vi "DatabaseToSharedVariable.vi"(8 "error in":errorcluster, 9 "database":string[][](array[string]), 11 "Library in":refnum<vi>) -> (0 "error out":errorcluster, 2 "Boolean":bool, 3 "Library out":refnum<vi>)   [LabVIEW 2014]
doc: "<B>Copyright</B>: (c) 2015 MHWirth. All rights reserved.\n\nThis subVI creates and addes shared variables to the given library. \nTo generate shared variables, it requires a 2D array of strings, whose first column contains the names and the second one contains the data type.\n\n<B>Limitation</B>: Not available in Run-time Engine."
panel:
  out "Numeric":i32
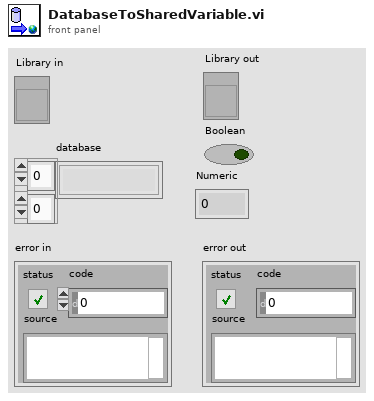
[diagram p1: front panel]
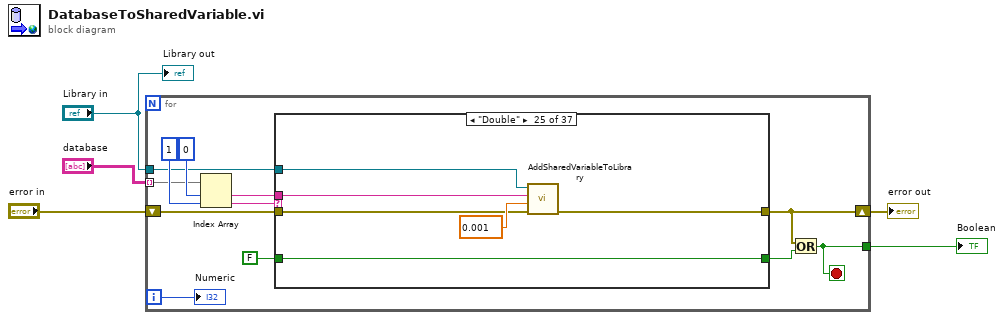
[diagram p0: block diagram]
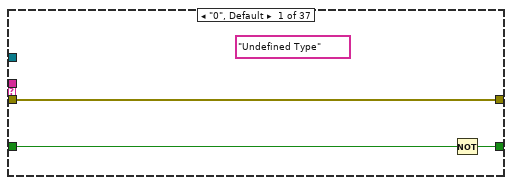
[diagram p2: hidden frame]
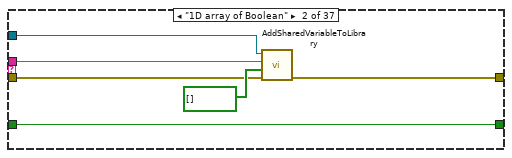
[diagram p3: hidden frame]
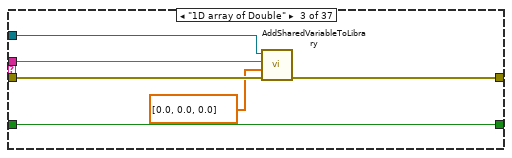
[diagram p4: hidden frame]
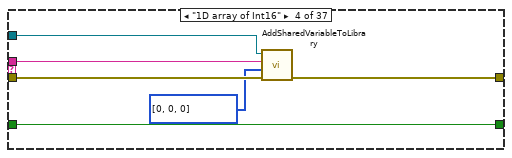
[diagram p5: hidden frame]
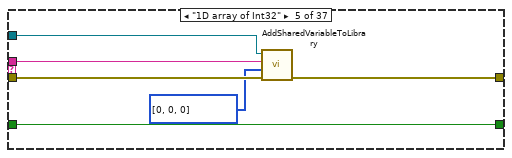
[diagram p6: hidden frame]
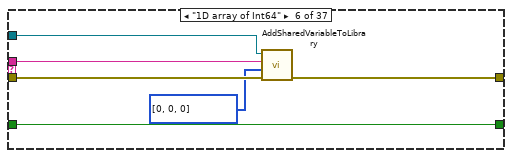
[diagram p7: hidden frame]
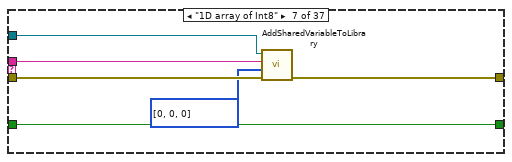
[diagram p8: hidden frame]
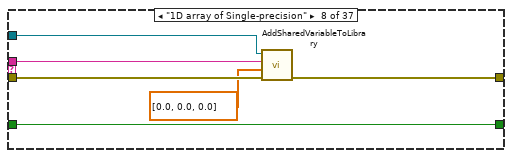
[diagram p9: hidden frame]
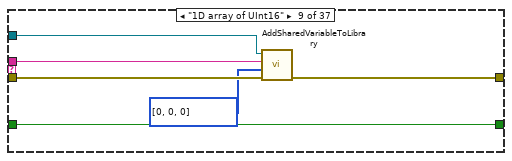
[diagram p10: hidden frame]
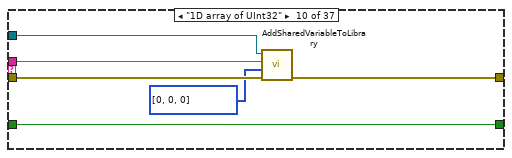
[diagram p11: hidden frame]
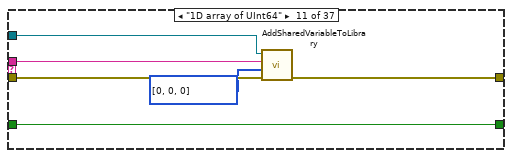
[diagram p12: hidden frame]
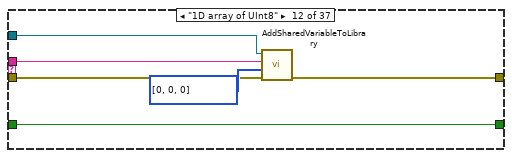
[diagram p13: hidden frame]
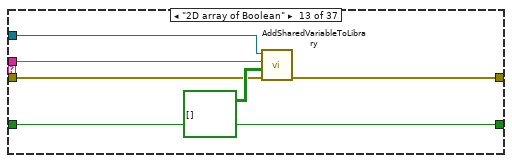
[diagram p14: hidden frame]
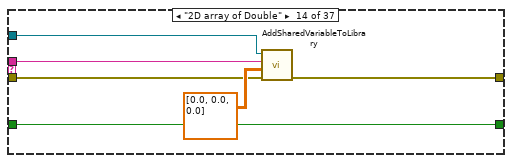
[diagram p15: hidden frame]
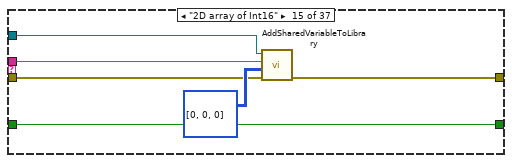
[diagram p16: hidden frame]
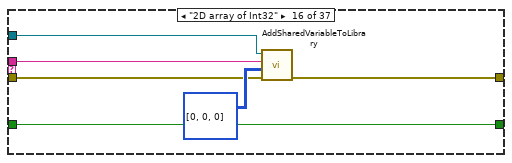
[diagram p17: hidden frame]
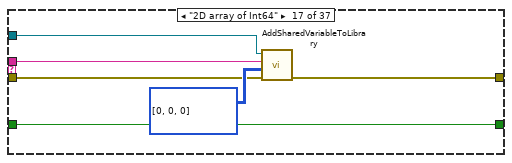
[diagram p18: hidden frame]
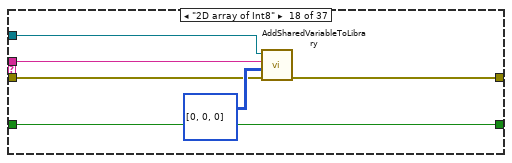
[diagram p19: hidden frame]
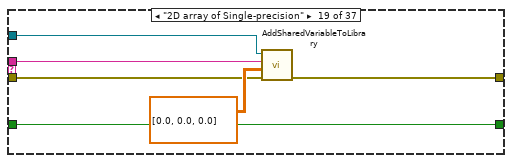
[diagram p20: hidden frame]
diagram:
  n1 = for {
    shift-right: [w7] -> w5
    shift-left: "error in" -> [w8]
    tunnel: "database" -> [w15] mode=indexing
    tunnel: [w11] -> w4
    tunnel: "Library in" -> [w9]
    i -> [w6]
    stop <- w11 stop-if-true
    n2 = Index Array(array=w15, index #1=0 ("index"), index #2=1 ("index")) -> (element #1=w10:string, element #2=w14:string)
    n3 = case shown="\"Double\"" w14 {
      tunnel: FALSE -> [w20 w26 w32 w38 w44 w50 w56 w62 w68 w74 w80 w86 w92 w98 w104 w110 w116 w122 w128 w134 w140 w146 w152 w158 w164 w170 w176 w182 w188 w194 w200 w206 w212 w218 w224 w230 w236]
      tunnel: [w19 w26 w32 w38 w44 w50 w56 w62 w68 w74 w80 w86 w92 w98 w104 w110 w116 w122 w128 w134 w140 w146 w152 w158 w164 w170 w176 w182 w188 w194 w200 w206 w212 w218 w224 w230 w236] -> w12
      tunnel: w10 -> [_ w25 w29 w34 w40 w47 w52 w58 w64 w70 w76 w82 w90 w95 w102 w108 w114 w120 w126 w131 w138 w144 w150 w156 w162 w167 w172 w180 w186 w192 w198 w204 w210 w216 w222 w228 w234]
      tunnel: w9 -> [_ w23 w28 w35 w43 w48 w51 w57 w65 w71 w75 w84 w91 w96 w103 w109 w115 w121 w127 w132 w139 w145 w151 w157 w163 w168 w173 w181 w187 w193 w199 w205 w211 w217 w223 w229 w235]
      tunnel: w8 -> [w18 w22 w30 w36 w42 w49 w54 w60 w66 w72 w78 w83 w88 w93 w100 w106 w112 w118 w124 w133 w136 w142 w148 w154 w160 w166 w174 w178 w184 w190 w196 w202 w208 w214 w220 w226 w232]
      tunnel: [w18 w21 w31 w37 w41 w45 w55 w61 w67 w73 w79 w81 w87 w97 w99 w105 w111 w117 w123 w129 w135 w141 w147 w153 w159 w165 w175 w177 w183 w189 w195 w201 w207 w213 w219 w225 w231] -> w7
      frame "0", Default {
        (unwired) "Undefined Type"
        n4 = Not(x=w20) -> (.not. x?=w19:bool)
      }
      frame "1D array of Boolean" {
        n5 = call <vilib>:"AddSharedVariableToLibrary.vi"("error in (no error)"=w22, "Variable Data Type (Double)"=bool[] [], "Variable Name"=w25, "Library Reference In"=w23) -> ("error out"=w21:errorcluster)  [unwired: 5 in, 2 out]
      }
      frame "1D array of Double" {
        n6 = call <vilib>:"AddSharedVariableToLibrary.vi"("error in (no error)"=w30, "Variable Data Type (Double)"=dbl[] [0.0, 0.0, 0.0], "Variable Name"=w29, "Library Reference In"=w28) -> ("error out"=w31:errorcluster)  [unwired: 5 in, 2 out]
      }
      frame "1D array of Int16" {
        n7 = call <vilib>:"AddSharedVariableToLibrary.vi"("error in (no error)"=w36, "Variable Data Type (Double)"=i16[] [0, 0, 0], "Variable Name"=w34, "Library Reference In"=w35) -> ("error out"=w37:errorcluster)  [unwired: 5 in, 2 out]
      }
      frame "1D array of Int32" {
        n8 = call <vilib>:"AddSharedVariableToLibrary.vi"("error in (no error)"=w42, "Variable Data Type (Double)"=i32[] [0, 0, 0], "Variable Name"=w40, "Library Reference In"=w43) -> ("error out"=w41:errorcluster)  [unwired: 5 in, 2 out]
      }
      frame "1D array of Int64" {
        n9 = call <vilib>:"AddSharedVariableToLibrary.vi"("error in (no error)"=w49, "Variable Data Type (Double)"=i64[] [0, 0, 0], "Variable Name"=w47, "Library Reference In"=w48) -> ("error out"=w45:errorcluster)  [unwired: 5 in, 2 out]
      }
      frame "1D array of Int8" {
        n10 = call <vilib>:"AddSharedVariableToLibrary.vi"("error in (no error)"=w54, "Variable Data Type (Double)"=i8[] [0, 0, 0], "Variable Name"=w52, "Library Reference In"=w51) -> ("error out"=w55:errorcluster)  [unwired: 5 in, 2 out]
      }
      frame "1D array of Single-precision" {
        n11 = call <vilib>:"AddSharedVariableToLibrary.vi"("error in (no error)"=w60, "Variable Data Type (Double)"=sgl[] [0.0, 0.0, 0.0], "Variable Name"=w58, "Library Reference In"=w57) -> ("error out"=w61:errorcluster)  [unwired: 5 in, 2 out]
      }
      frame "1D array of UInt16" {
        n12 = call <vilib>:"AddSharedVariableToLibrary.vi"("error in (no error)"=w66, "Variable Data Type (Double)"=u16[] [0, 0, 0], "Variable Name"=w64, "Library Reference In"=w65) -> ("error out"=w67:errorcluster)  [unwired: 5 in, 2 out]
      }
      frame "1D array of UInt32" {
        n13 = call <vilib>:"AddSharedVariableToLibrary.vi"("error in (no error)"=w72, "Variable Data Type (Double)"=u32[] [0, 0, 0], "Variable Name"=w70, "Library Reference In"=w71) -> ("error out"=w73:errorcluster)  [unwired: 5 in, 2 out]
      }
      frame "1D array of UInt64" {
        n14 = call <vilib>:"AddSharedVariableToLibrary.vi"("error in (no error)"=w78, "Variable Data Type (Double)"=u64[] [0, 0, 0], "Variable Name"=w76, "Library Reference In"=w75) -> ("error out"=w79:errorcluster)  [unwired: 5 in, 2 out]
      }
      frame "1D array of UInt8" {
        n15 = call <vilib>:"AddSharedVariableToLibrary.vi"("error in (no error)"=w83, "Variable Data Type (Double)"=u8[] [0, 0, 0], "Variable Name"=w82, "Library Reference In"=w84) -> ("error out"=w81:errorcluster)  [unwired: 5 in, 2 out]
      }
      frame "2D array of Boolean" {
        n16 = call <vilib>:"AddSharedVariableToLibrary.vi"("error in (no error)"=w88, "Variable Data Type (Double)"=bool[][] [], "Variable Name"=w90, "Library Reference In"=w91) -> ("error out"=w87:errorcluster)  [unwired: 5 in, 2 out]
      }
      frame "2D array of Double" {
        n17 = call <vilib>:"AddSharedVariableToLibrary.vi"("error in (no error)"=w93, "Variable Data Type (Double)"=dbl[][] [[0.0, 0.0, 0.0]], "Variable Name"=w95, "Library Reference In"=w96) -> ("error out"=w97:errorcluster)  [unwired: 5 in, 2 out]
      }
      frame "2D array of Int16" {
        n18 = call <vilib>:"AddSharedVariableToLibrary.vi"("error in (no error)"=w100, "Variable Data Type (Double)"=i16[][] [[0, 0, 0]], "Variable Name"=w102, "Library Reference In"=w103) -> ("error out"=w99:errorcluster)  [unwired: 5 in, 2 out]
      }
      frame "2D array of Int32" {
        n19 = call <vilib>:"AddSharedVariableToLibrary.vi"("error in (no error)"=w106, "Variable Data Type (Double)"=i32[][] [[0, 0, 0]], "Variable Name"=w108, "Library Reference In"=w109) -> ("error out"=w105:errorcluster)  [unwired: 5 in, 2 out]
      }
      frame "2D array of Int64" {
        n20 = call <vilib>:"AddSharedVariableToLibrary.vi"("error in (no error)"=w112, "Variable Data Type (Double)"=i64[][] [[0, 0, 0]], "Variable Name"=w114, "Library Reference In"=w115) -> ("error out"=w111:errorcluster)  [unwired: 5 in, 2 out]
      }
      frame "2D array of Int8" {
        n21 = call <vilib>:"AddSharedVariableToLibrary.vi"("error in (no error)"=w118, "Variable Data Type (Double)"=i8[][] [[0, 0, 0]], "Variable Name"=w120, "Library Reference In"=w121) -> ("error out"=w117:errorcluster)  [unwired: 5 in, 2 out]
      }
      frame "2D array of Single-precision" {
        n22 = call <vilib>:"AddSharedVariableToLibrary.vi"("error in (no error)"=w124, "Variable Data Type (Double)"=sgl[][] [[0.0, 0.0, 0.0]], "Variable Name"=w126, "Library Reference In"=w127) -> ("error out"=w123:errorcluster)  [unwired: 5 in, 2 out]
      }
      frame "2D array of UInt16" {
        n23 = call <vilib>:"AddSharedVariableToLibrary.vi"("error in (no error)"=w133, "Variable Data Type (Double)"=u16[][] [[0, 0, 0]], "Variable Name"=w131, "Library Reference In"=w132) -> ("error out"=w129:errorcluster)  [unwired: 5 in, 2 out]
      }
      frame "2D array of UInt32" {
        n24 = call <vilib>:"AddSharedVariableToLibrary.vi"("error in (no error)"=w136, "Variable Data Type (Double)"=u32[][] [[0, 0, 0]], "Variable Name"=w138, "Library Reference In"=w139) -> ("error out"=w135:errorcluster)  [unwired: 5 in, 2 out]
      }
      frame "2D array of UInt64" {
        n25 = call <vilib>:"AddSharedVariableToLibrary.vi"("error in (no error)"=w142, "Variable Data Type (Double)"=u64[][] [[0, 0, 0]], "Variable Name"=w144, "Library Reference In"=w145) -> ("error out"=w141:errorcluster)  [unwired: 5 in, 2 out]
      }
      frame "2D array of UInt8" {
        n26 = call <vilib>:"AddSharedVariableToLibrary.vi"("error in (no error)"=w148, "Variable Data Type (Double)"=u8[][] [[0, 0, 0]], "Variable Name"=w150, "Library Reference In"=w151) -> ("error out"=w147:errorcluster)  [unwired: 5 in, 2 out]
      }
      frame "Boolean" {
        n27 = call <vilib>:"AddSharedVariableToLibrary.vi"("error in (no error)"=w154, "Variable Data Type (Double)"=FALSE, "Variable Name"=w156, "Library Reference In"=w157) -> ("error out"=w153:errorcluster)  [unwired: 5 in, 2 out]
      }
      frame "Double" {
        n28 = call <vilib>:"AddSharedVariableToLibrary.vi"("error in (no error)"=w160, "Variable Data Type (Double)"=0.001, "Variable Name"=w162, "Library Reference In"=w163) -> ("error out"=w159:errorcluster)  [unwired: 5 in, 2 out]
      }
      frame "Fixed Point - signed" {
        n29 = call <vilib>:"AddSharedVariableToLibrary.vi"("error in (no error)"=w166, "Variable Data Type (Double)"=fxp<+/-,32,16> 0.001007080078125, "Variable Name"=w167, "Library Reference In"=w168) -> ("error out"=w165:errorcluster)  [unwired: 5 in, 2 out]
      }
      frame "Fixed Point - unsigned" {
        n30 = call <vilib>:"AddSharedVariableToLibrary.vi"("error in (no error)"=w174, "Variable Data Type (Double)"=fxp<+,32,16> 0.001007080078125, "Variable Name"=w172, "Library Reference In"=w173) -> ("error out"=w175:errorcluster)  [unwired: 5 in, 2 out]
      }
      frame "Int16" {
        n31 = call <vilib>:"AddSharedVariableToLibrary.vi"("error in (no error)"=w178, "Variable Data Type (Double)"=i16 0, "Variable Name"=w180, "Library Reference In"=w181) -> ("error out"=w177:errorcluster)  [unwired: 5 in, 2 out]
      }
      frame "Int32" {
        n32 = call <vilib>:"AddSharedVariableToLibrary.vi"("error in (no error)"=w184, "Variable Data Type (Double)"=0, "Variable Name"=w186, "Library Reference In"=w187) -> ("error out"=w183:errorcluster)  [unwired: 5 in, 2 out]
      }
      frame "Int64" {
        n33 = call <vilib>:"AddSharedVariableToLibrary.vi"("error in (no error)"=w190, "Variable Data Type (Double)"=i64 0, "Variable Name"=w192, "Library Reference In"=w193) -> ("error out"=w189:errorcluster)  [unwired: 5 in, 2 out]
      }
      frame "Int8" {
        n34 = call <vilib>:"AddSharedVariableToLibrary.vi"("error in (no error)"=w196, "Variable Data Type (Double)"=i8 0, "Variable Name"=w198, "Library Reference In"=w199) -> ("error out"=w195:errorcluster)  [unwired: 5 in, 2 out]
      }
      frame "Single-precision" {
        n35 = call <vilib>:"AddSharedVariableToLibrary.vi"("error in (no error)"=w202, "Variable Data Type (Double)"=sgl 0.001, "Variable Name"=w204, "Library Reference In"=w205) -> ("error out"=w201:errorcluster)  [unwired: 5 in, 2 out]
      }
      frame "UInt16" {
        n36 = call <vilib>:"AddSharedVariableToLibrary.vi"("error in (no error)"=w208, "Variable Data Type (Double)"=u16 0, "Variable Name"=w210, "Library Reference In"=w211) -> ("error out"=w207:errorcluster)  [unwired: 5 in, 2 out]
      }
      frame "UInt32" {
        n37 = call <vilib>:"AddSharedVariableToLibrary.vi"("error in (no error)"=w214, "Variable Data Type (Double)"=u32 0, "Variable Name"=w216, "Library Reference In"=w217) -> ("error out"=w213:errorcluster)  [unwired: 5 in, 2 out]
      }
      frame "UInt64" {
        n38 = call <vilib>:"AddSharedVariableToLibrary.vi"("error in (no error)"=w220, "Variable Data Type (Double)"=u64 0, "Variable Name"=w222, "Library Reference In"=w223) -> ("error out"=w219:errorcluster)  [unwired: 5 in, 2 out]
      }
      frame "UInt8" {
        n39 = call <vilib>:"AddSharedVariableToLibrary.vi"("error in (no error)"=w226, "Variable Data Type (Double)"=u8 0, "Variable Name"=w228, "Library Reference In"=w229) -> ("error out"=w225:errorcluster)  [unwired: 5 in, 2 out]
      }
      frame "String" {
        n40 = call <vilib>:"AddSharedVariableToLibrary.vi"("error in (no error)"=w232, "Variable Data Type (Double)"="a", "Variable Name"=w234, "Library Reference In"=w235) -> ("error out"=w231:errorcluster)  [unwired: 5 in, 2 out]
      }
    }
    n41 = Or(x=w7, y=w12) -> (x .or. y?=w11:bool)
    "Numeric" <- w6
  }
  "error out" <- w5
  "Boolean" <- w4
  "Library out" <- "Library in"
